vi "MCA Display.vi"(8 "error in (no error)":errorcluster, 9 "Module number":u16, 10 "stop":bool, 11 "channel":string(combo)) -> (0 "error out":errorcluster, 1 "raw histo":u32[](array[numeric]), 2 "stop out":bool, 3 "MCA Histograms":u32[][](graph))   [LabVIEW 2016]
doc: "Displays 1d spectrum from internal pixie memory"
uses:
  Drivers/Pixie4DLL.dll
panel:
  out "sum 4":u32
  out "sum 3":u32
  out "sum 2":u32
  out "sum":u32
  out "channel 1/ eres":dbl
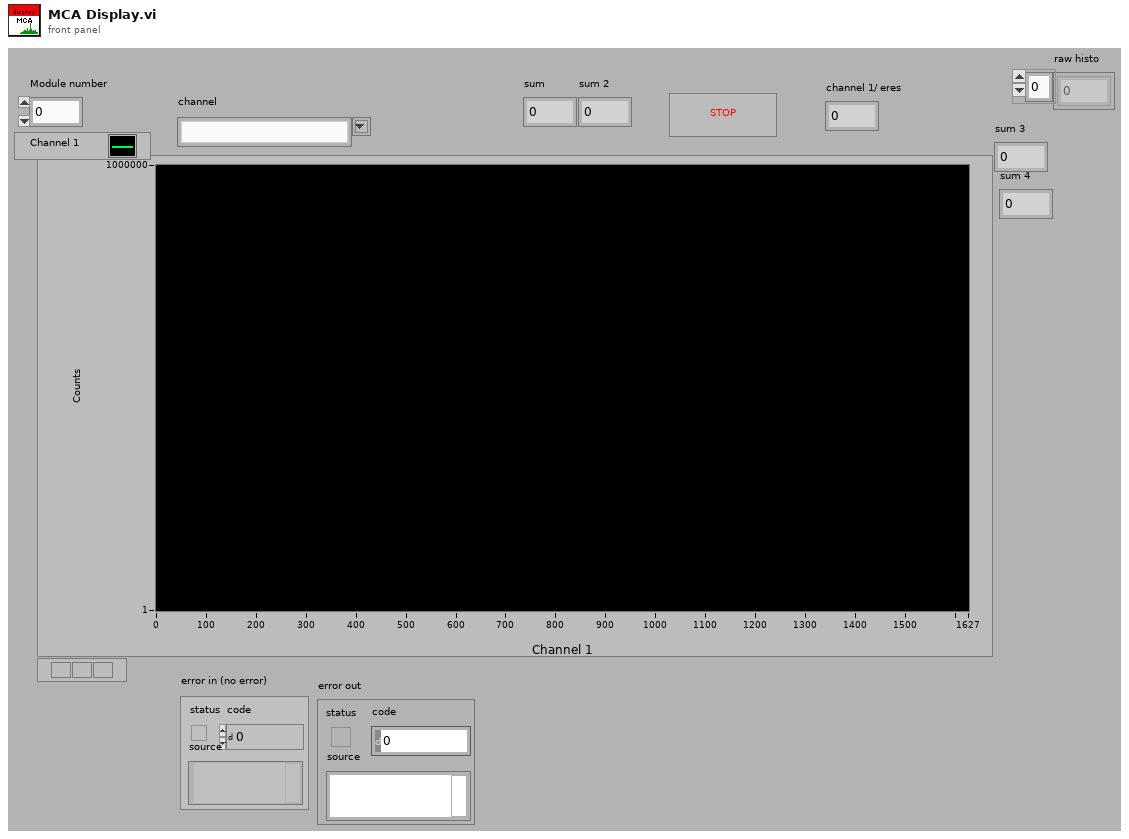
[diagram p1: front panel]
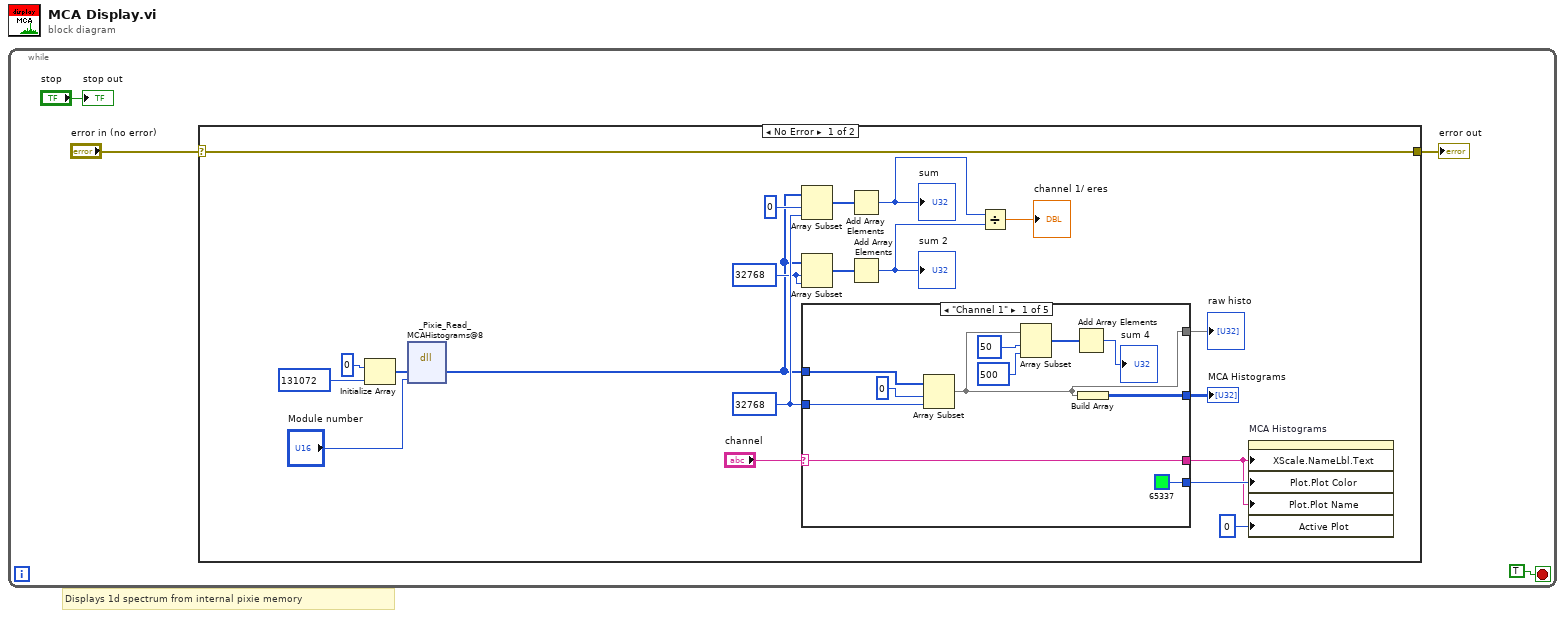
[diagram p0: block diagram]
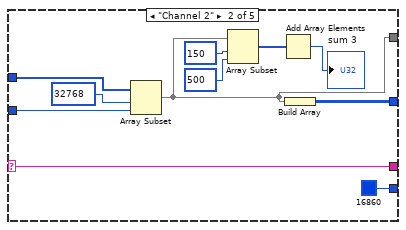
[diagram p2: hidden frame]
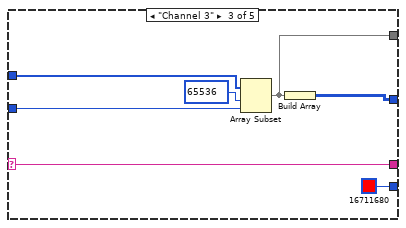
[diagram p3: hidden frame]
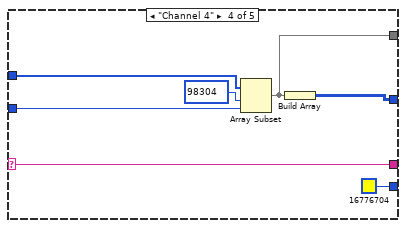
[diagram p4: hidden frame]
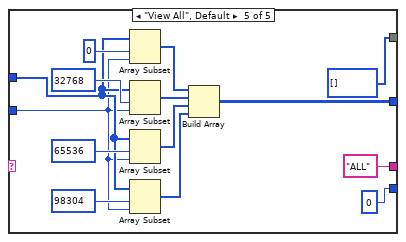
[diagram p5: hidden frame]
diagram:
  # "Displays 1d spectrum from internal pixie memory"
  n1 = while {
    stop <- TRUE stop-if-true
    n2 = case shown="No Error" "error in (no error)" {
      selector: "error in (no error)" -> [w18 w75]
      tunnel: [w18 w75] -> w2
      frame No Error {
        w13 = 32768
        w14 = 32768
        n3 = Initialize Array(0, 131072) -> (w23:i32[])
        n4 = dll-call lib="D:/Users/wymanm/Desktop/DAQuiri - 2017a/lois/Drivers/Pixie4DLL.dll" fn="_Pixie_Read_MCAHistograms@8"("MCAHistograms"=w23, "ModNum"="Module number") -> ("MCAHistograms"=w6:u32[])  [unwired: 5 in, 2 out]
        n5 = Array Subset(array=w6, index=0, length=w14) -> (w12:u32[])
        n6 = Array Subset(array=w6, index=w13, length=w13) -> (w11:u32[])
        n7 = case shown="\"Channel 1\"" "channel" {
          selector: "channel" -> [w30 w42 w49 w56 _]
          tunnel: w14 -> [w34 w45 w52 w59 w65]
          tunnel: w6 -> [w33 w44 w51 w58 w66]
          tunnel: [w32 w43 w50 w57 w64] -> w7
          tunnel: [w30 w42 w49 w56 "ALL"] -> w16
          tunnel: [u32 65337 ("Color Box") u32 16860 ("Color Box") u32 16711680 ("Color Box") u32 16776704 ("Color Box") u32 0 ("Color Box")] -> w19
          tunnel: [w25 w36 w47 w54 u32[] []] -> w5
          frame "Channel 1" {
            n8 = Array Subset(array=w33, index=0, length=w34) -> (w25:u32[])
            n9 = Array Subset(array=w25, index=50, length=500) -> (w27:u32[])
            n10 = Add Array Elements(numeric array=w27) -> (sum=→"sum 4":u32)
            n11 = Build Array(w25) -> (w32:u32[][])
          }
          frame "Channel 2" {
            n12 = Array Subset(array=w44, index=32768, length=w45) -> (w36:u32[])
            n13 = Array Subset(array=w36, index=150, length=500) -> (w38:u32[])
            n14 = Add Array Elements(numeric array=w38) -> (sum=→"sum 3":u32)
            n15 = Build Array(w36) -> (w43:u32[][])
          }
          frame "Channel 3" {
            n16 = Array Subset(array=w51, index=65536, length=w52) -> (w47:u32[])
            n17 = Build Array(w47) -> (w50:u32[][])
          }
          frame "Channel 4" {
            n18 = Array Subset(array=w58, index=98304, length=w59) -> (w54:u32[])
            n19 = Build Array(w54) -> (w57:u32[][])
          }
          frame "View All", Default {
            n20 = Array Subset(array=w66, index=0, length=w65) -> (w69:u32[])
            n21 = Array Subset(array=w66, index=32768, length=w65) -> (w68:u32[])
            n22 = Array Subset(array=w66, index=65536, length=w65) -> (w74:u32[])
            n23 = Array Subset(array=w66, index=98304, length=w65) -> (w67:u32[])
            n24 = Build Array(w69, w68, w74, w67) -> (w64:u32[][])
          }
        }
        "MCA Histograms" <- w7
        "raw histo" <- w5
        n25 = Add Array Elements(numeric array=w12) -> (sum=w9:u32)
        "sum" <- w9
        n26 = Add Array Elements(numeric array=w11) -> (sum=w10:u32)
        "sum 2" <- w10
        n27 = Divide(x=w9, y=w10) -> (x/y=→"channel 1/ eres":dbl)
        n28 = property on="MCA Histograms" class="WFGraph (strict)"("XScale.NameLbl.Text"=w16, "Plot.Plot Color"=w19, "Plot.Plot Name"=w16, "Active Plot"=u32 0) -> ()  [unwired: 2 in, 2 out]
      }
      frame Error {
      }
    }
    "error out" <- w2
    "stop out" <- "stop"
  }
